vi "Remote PC - Client_DUT1.vi"(0 "IP Address":string="localhost", 2 "Flow Contorl":enum16{"Connect", "Read", "Write", "Close"}(ring)=enum."Write", 5 "Log Path":path=path "D:/My Projects/MitraStar/wlan test lib - onsite - second round/Report SubVIs/DUT 1_9_09_38 AM 10_24_2013_Report.csv", 7 "Send Command":T1="Analyze Log", 9 "ServerTCPhandle":refnum<k5>, 11 "error in":errorcluster, 12 "Remote Sever Port (2800)":u16) -> (4 "MAC&SN":string, 6 "TCPHandle":refnum<k5>, 10 "Receive Message":string, 15 "error out":errorcluster)   [LabVIEW 2012]
uses:
  TypeDef/Send Command Message.ctl
panel:
  out "concatenated string":string
  out "bytes written":i32=19538
  out "data out":string="DONE\r\n"
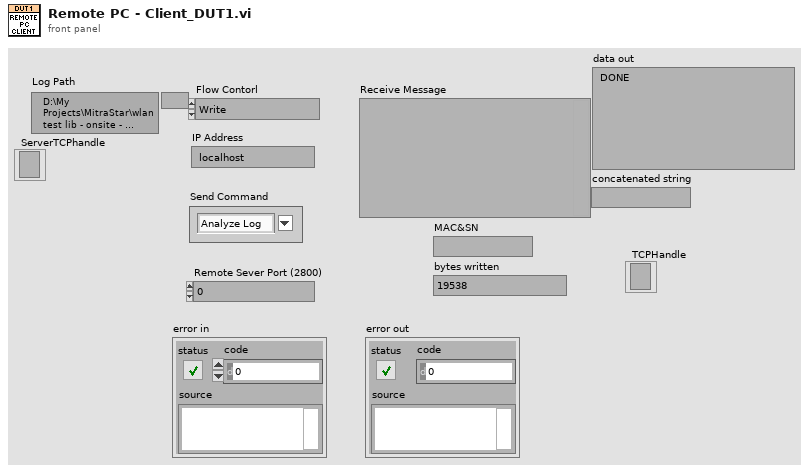
[diagram p1: front panel]
types:
  T1 = typedef "Send Command Message.ctl" = string
  T2 = enum16{"Standard", "Buffered", "CRLF", "Immediate"}
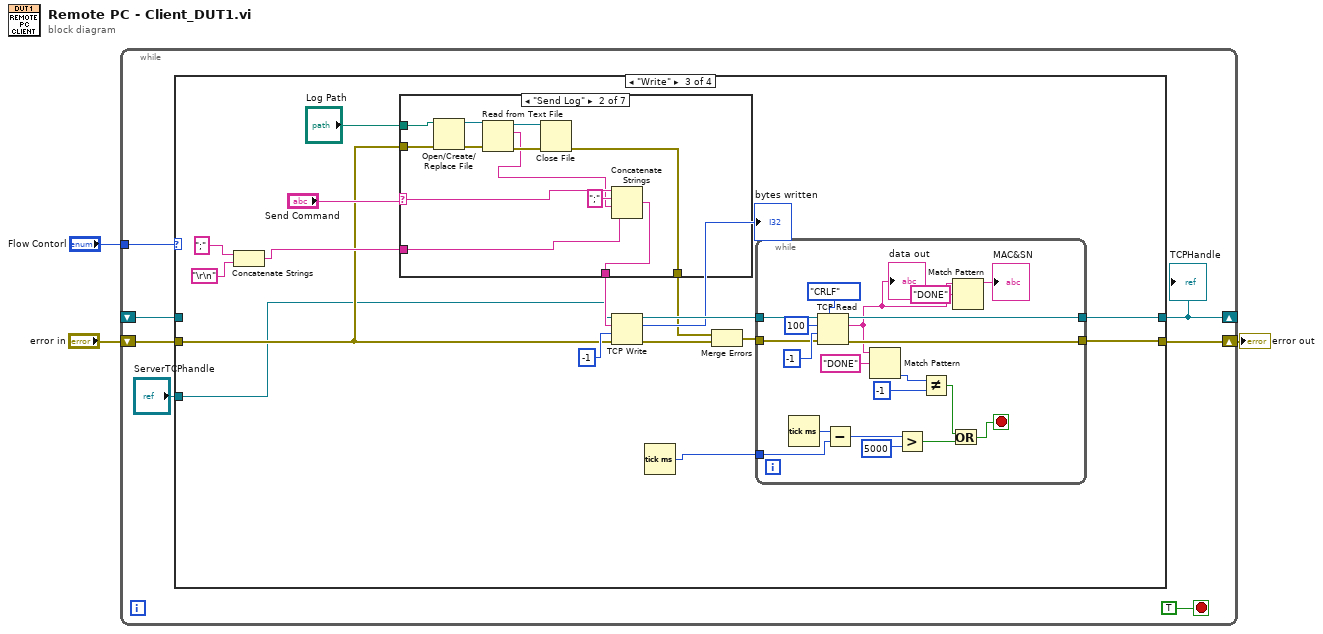
[diagram p0: block diagram]
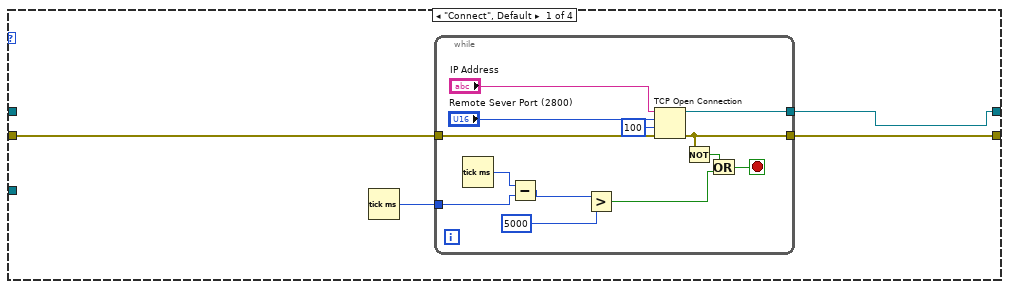
[diagram p2: hidden frame]
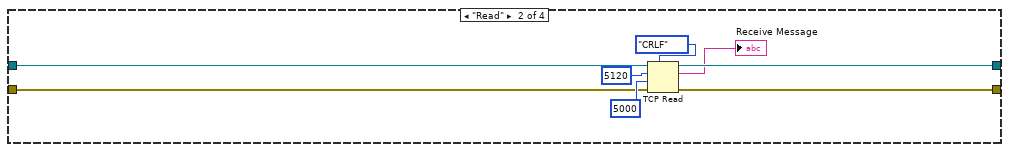
[diagram p3: hidden frame]
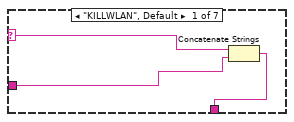
[diagram p4: hidden frame]
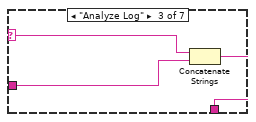
[diagram p5: hidden frame]
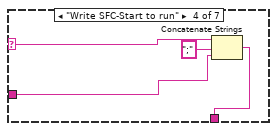
[diagram p6: hidden frame]
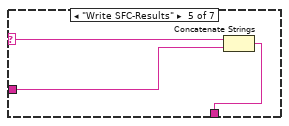
[diagram p7: hidden frame]
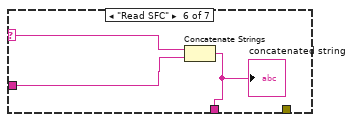
[diagram p8: hidden frame]
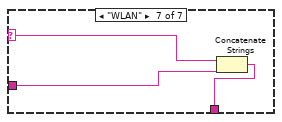
[diagram p9: hidden frame]
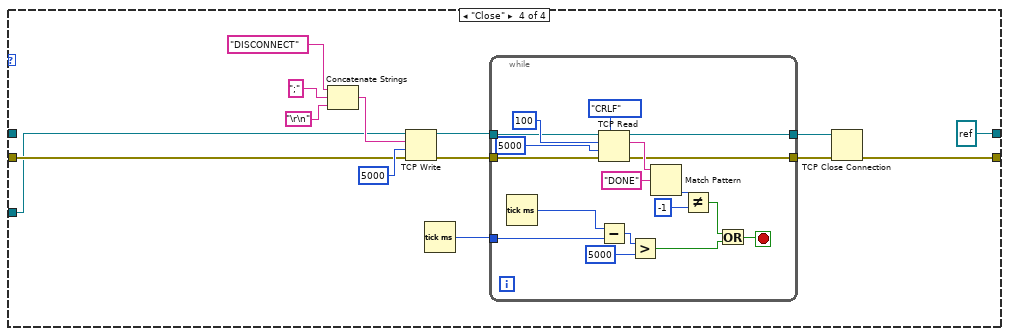
[diagram p10: hidden frame]
diagram:
  n1 = while {
    shift-right: [w8] -> w2
    shift-left: "error in" -> [w9]
    shift-right: [w4] -> _
    shift-left: _ -> [w7]
    tunnel: "Flow Contorl" -> [w6]
    stop <- TRUE stop-if-true
    n2 = case shown="\"Write\"" w6 {
      tunnel: w9 -> [w14 w31 w40 w114]
      tunnel: [w13 w30 w49 w117] -> w8
      tunnel: [w11 w29 w50 refnum<k5> refnum ("connection ID")] -> w4
      tunnel: w7 -> [_ w32 _ _]
      tunnel: "ServerTCPhandle" -> [_ _ w36 w104]
      frame "Connect", Default {
        n3 = Tick Count (ms)() -> (millisecond timer value=w12:u32)
        n4 = while {
          tunnel: w14 -> [w25]
          tunnel: [w16] -> w13
          tunnel: [w24] -> w11
          tunnel: w12 -> [w21]
          stop <- w17 stop-if-true
          n5 = Tick Count (ms)() -> (millisecond timer value=w22:u32)
          n6 = Subtract(x=w22, y=w21) -> (x-y=w20:u32)
          n7 = Greater?(x=w20, y=u32 5000) -> (0:w18:bool)
          n8 = TCP Open Connection(address="IP Address", remote port or service name="Remote Sever Port (2800)", timeout ms (60000)=100, error in (no error)=w25) -> (connection ID=w24:refnum<k5>, error out=w16:errorcluster)  [unwired: 1 in]
          n9 = Not(x=w16) -> (.not. x?=w15:bool)
          n10 = Or(x=w15, y=w18) -> (x .or. y?=w17:bool)
        }
      }
      frame "Read" {
        n11 = TCP Read(connection ID=w32, bytes to read=5120, error in (no error)=w31, 7:T2."CRLF" ("mode (standard)"), 9:5000 ("timeout ms (25000)")) -> (connection ID out=w29:refnum<k5>, data out=→"Receive Message":string, error out=w30:errorcluster)
      }
      frame "Write" {
        n12 = Concatenate Strings(";", "\r\n") -> (w44:string)
        n13 = case shown="\"Send Log\"" "Send Command" {
          selector: "Send Command" -> [w55 w66 w70 w73 w77 w80 w83]
          tunnel: [w54 w67 w69 w74 w75 w79 w82] -> w47
          tunnel: w44 -> [w53 w64 w68 w71 w76 w78 w81]
          tunnel: "Log Path" -> [_ w58 _ _ _ _ _]
          tunnel: w40 -> [_ w57 _ _ _ _ _]
          tunnel: [_ w56 _ _ _ _ _] -> w37
          frame "KILLWLAN", Default {
            n14 = Concatenate Strings(w55, w53) -> (w54:string)
          }
          frame "Send Log" {
            n15 = Open/Create/Replace File(file path (use dialog)=w58, error in=w57) -> (refnum out=w61:refnum<file>, error out=w60:errorcluster)  [unwired: 4 in, 1 out]
            n16 = Read from Text File(file (use dialog)=w61, error in=w60) -> (refnum out=w63:refnum<file>, text=w59:string, error out=w62:errorcluster)  [unwired: 2 in, 1 out]
            n17 = Close File(refnum=w63, error in=w62) -> (error out=w56:errorcluster)  [unwired: 1 out]
            n18 = Concatenate Strings(w66, ";" ("string"), w59, w64) -> (w67:string)
          }
          frame "Analyze Log" {
            n19 = Concatenate Strings(w70, w68) -> (w69:string)
          }
          frame "Write SFC-Start to run" {
            n20 = Concatenate Strings(w73, ";" ("string"), w71) -> (w74:string)
          }
          frame "Write SFC-Results" {
            n21 = Concatenate Strings(w77, w76) -> (w75:string)
          }
          frame "Read SFC" {
            n22 = Concatenate Strings(w80, w78) -> (w79:string)
            "concatenated string" <- w79
          }
          frame "WLAN" {
            n23 = Concatenate Strings(w83, w81) -> (w82:string)
          }
        }
        n24 = TCP Write(connection ID=w36, data in=w47, error in (no error)=w40, 9:-1 ("timeout ms (25000)")) -> (connection ID out=w51:refnum<k5>, bytes written=→"bytes written":i32, error out=w39:errorcluster)
        n25 = Tick Count (ms)() -> (millisecond timer value=w41:u32)
        n26 = Merge Errors(w37, w39) -> (w38:errorcluster)
        n27 = while {
          tunnel: [w97] -> w50
          tunnel: [w96] -> w49
          tunnel: w51 -> [w95]
          tunnel: w38 -> [w94]
          tunnel: w41 -> [w89]
          stop <- w84 stop-if-true
          n28 = Tick Count (ms)() -> (millisecond timer value=w90:u32)
          n29 = TCP Read(connection ID=w95, bytes to read=100, error in (no error)=w94, 7:T2."CRLF" ("mode (standard)"), 9:-1 ("timeout ms (25000)")) -> (connection ID out=w97:refnum<k5>, data out=w93:string, error out=w96:errorcluster)
          "data out" <- w93
          n30 = Subtract(x=w90, y=w89) -> (x-y=w88:u32)
          n31 = Match Pattern(string=w93, regular expression="DONE") -> (offset past match=w100:i32)  [unwired: 1 in, 3 out]
          n32 = Greater?(x=w88, y=u32 5000) -> (0:w86:bool)
          n33 = Not Equal?(x=w100, y=-1) -> (x != y?=w85:bool)
          n34 = Or(x=w85, y=w86) -> (x .or. y?=w84:bool)
          n35 = Match Pattern(string=w93, regular expression="DONE") -> (before substring=→"MAC&SN":string)  [unwired: 1 in, 3 out]
        }
      }
      frame "Close" {
        n36 = Concatenate Strings("DISCONNECT" ("data in"), ";", "\r\n") -> (w105:string)
        n37 = TCP Write(connection ID=w104, data in=w105, error in (no error)=w114, 9:5000 ("timeout ms (25000)")) -> (connection ID out=w110:refnum<k5>, error out=w109:errorcluster)  [unwired: 1 out]
        n38 = Tick Count (ms)() -> (millisecond timer value=w113:u32)
        n39 = while {
          tunnel: w113 -> [w127]
          tunnel: [w121] -> w112
          tunnel: [w120] -> w111
          tunnel: w110 -> [w119]
          tunnel: w109 -> [w118]
          stop <- w122 stop-if-true
          n40 = Tick Count (ms)() -> (millisecond timer value=w128:u32)
          n41 = TCP Read(connection ID=w119, bytes to read=100, error in (no error)=w118, 7:T2."CRLF" ("mode (standard)"), 9:5000 ("timeout ms (25000)")) -> (connection ID out=w121:refnum<k5>, data out=w133:string, error out=w120:errorcluster)
          n42 = Subtract(x=w128, y=w127) -> (x-y=w126:u32)
          n43 = Greater?(x=w126, y=u32 5000) -> (0:w123:bool)
          n44 = Match Pattern(string=w133, regular expression="DONE") -> (offset past match=w131:i32)  [unwired: 1 in, 3 out]
          n45 = Not Equal?(x=w131, y=-1) -> (x != y?=w124:bool)
          n46 = Or(x=w124, y=w123) -> (x .or. y?=w122:bool)
        }
        n47 = TCP Close Connection(connection ID=w112, error in (no error)=w111) -> (error out=w117:errorcluster)  [unwired: 1 in, 1 out]
      }
    }
    "TCPHandle" <- w4
  }
  "error out" <- w2
